vi "fgv_curr-test-info.vi"(7 "cmd":T3, 11 "현재테스트 정보":T1) -> (3 "현재테스트 정보 2":T1)   [LabVIEW 2019]
uses:
  _ctrl/rw.ctl
  _ctrl/Testing-info.ctl
  sequence_single.ctl
  SubVIs/common/Glob_Ref.vi
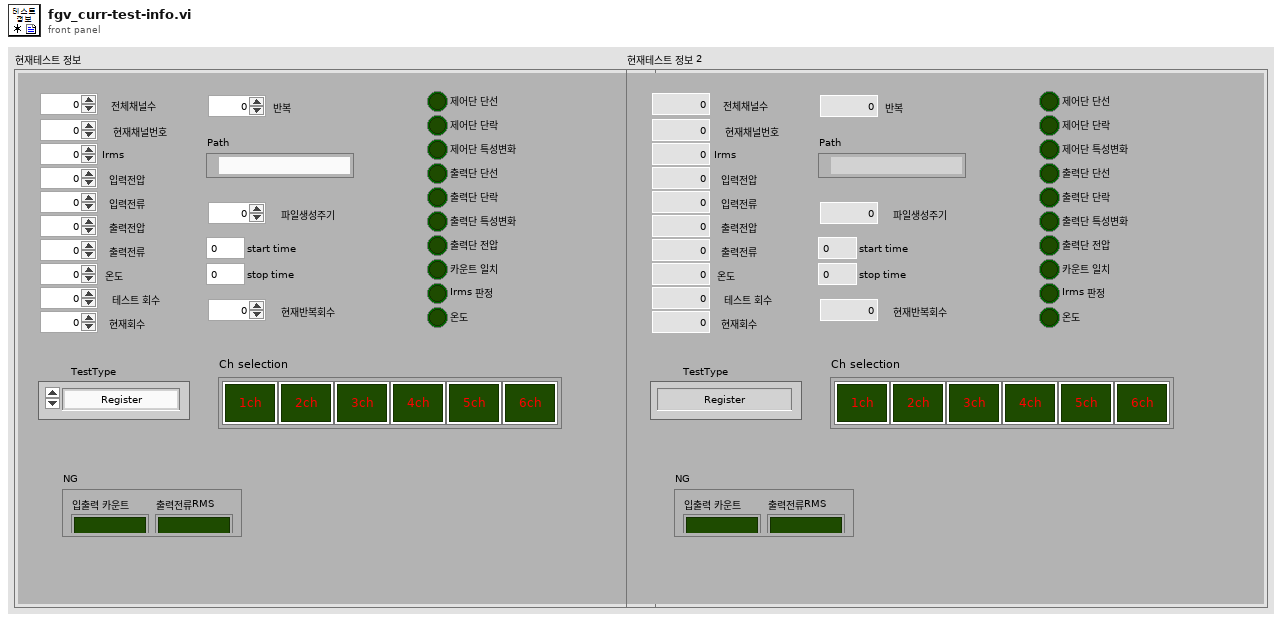
[diagram p1: front panel]
types:
  T1 = typedef "Testing-info.ctl" = cluster{"전체채널수":u8, "현재채널번호":u8, "Irms":dbl, "입력전압":dbl, "입력전류":dbl, "출력전압":dbl, "출력전류":dbl, "온도":dbl, "제어단 단선":bool, "제어단 단락":bool, "제어단 특성변화":bool, "출력단 단선":bool, "출력단 단락":bool, "출력단 특성변화":bool, "출력단 전압":bool, "카운트 일치":bool, "Irms 판정":bool, "온도":bool, "테스트 회수":u32, "TestType":T2, "현재회수":u32, "Ch selection":cluster{"1ch":bool, "2ch":bool, "3ch":bool, "4ch":bool, "5ch":bool, "6ch":bool}, "반복":u32, "Path":path, "파일생성주기":u32, "start time":dbl, "stop time":dbl, "현재반복회수":u32, "NG":cluster{"입출력 카운트":bool, "출력전류RMS":bool}}
  T2 = typedef "sequence_single.ctl" = enum16{"Register", "RC", "B1", "B2", "B3", "Oper_LV", "Oper_HV", "ContR_LV"}
  T3 = typedef "rw.ctl" = enum16{"read", "write"}
  T4 = typedef "UI dev-operator.ctl" = enum16{"Testing", "Admin", "Operator", "Finish", "Ready"}
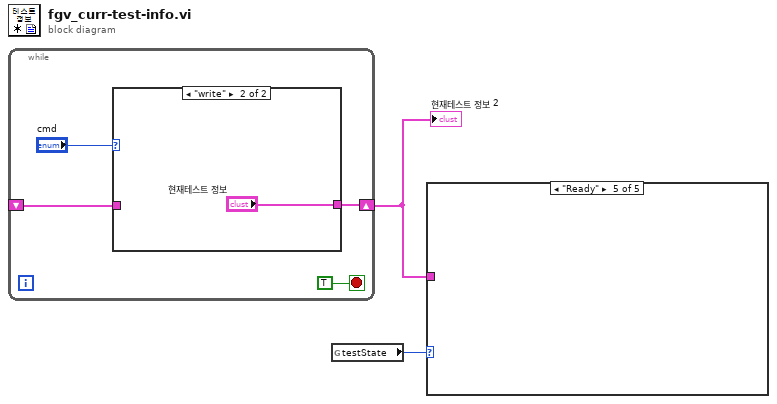
[diagram p0: block diagram]
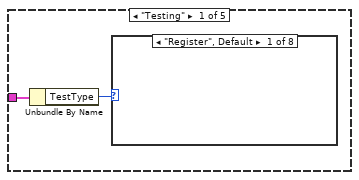
[diagram p2: hidden frame]
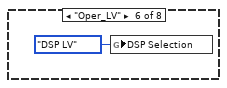
[diagram p7: hidden frame]
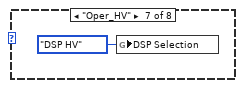
[diagram p8: hidden frame]
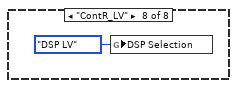
[diagram p9: hidden frame]
diagram:
  n1 = while {
    shift-right: [w4] -> w2
    shift-left: _ -> [w3]
    stop <- TRUE stop-if-true
    n2 = case shown="\"write\"" "cmd" {
      tunnel: [w7 "현재테스트 정보"] -> w4
      tunnel: w3 -> [w7 _]
      frame "read", Default {
      }
      frame "write" {
      }
    }
  }
  "현재테스트 정보 2" <- w2
  n3 = global read "Glob_Ref.vi" "testState"() -> (w1:T4)
  n4 = case shown="\"Ready\"" w1 {
    tunnel: w2 -> [w10 _ _ _ _]
    frame "Testing" {
      n5 = Unbundle By Name(w10) -> ("TestType"=w9:T2)
      n6 = case shown="\"Register\", Default" w9 {
        frame "Register", Default {
        }
        frame "RC" {
        }
        frame "B1" {
        }
        frame "B2" {
        }
        frame "B3" {
        }
        frame "Oper_LV" {
          n7 = global write "Glob_Ref.vi" "DSP Selection"(enum32{"DSP HV", "DSP LV"}."DSP LV" ("DSP Selection")) -> ()
        }
        frame "Oper_HV" {
          n8 = global write "Glob_Ref.vi" "DSP Selection"(enum32{"DSP HV", "DSP LV"}."DSP HV" ("DSP Selection")) -> ()
        }
        frame "ContR_LV" {
          n9 = global write "Glob_Ref.vi" "DSP Selection"(enum32{"DSP HV", "DSP LV"}."DSP LV" ("DSP Selection")) -> ()
        }
      }
    }
    frame "Admin" {
    }
    frame "Operator" {
    }
    frame "Finish", Default {
    }
    frame "Ready" {
    }
  }
